vi "readFromXML.vi"(8 "error in (no error)":errorcluster, 11 "file path (use dialog)":path) -> (0 "error out":errorcluster, 3 "Report (Ausgang)":refnum<class "Report.lvclass">)   [LabVIEW 2013, in "XML.lvlib"]
uses:
  lib/XML.lvlib
  classes/Datastructure/Report/Report.lvclass
  classes/Datastructure/Norm/Norm.lvclass
  classes/Datastructure/Test/Test.lvclass
  classes/Datastructure/Image/img.lvclass
  classes/Datastructure/Setup/Setup.lvclass
  classes/Datastructure/Device/Device.lvclass
  <vilib>/xml/Load XML File.vi
  <resource>/objmgr/DOMUserDefRef.rc
  <vilib>/xml/NI_XML.lvlib
panel:
  in  "img id":i32
  out "size(s)":i32
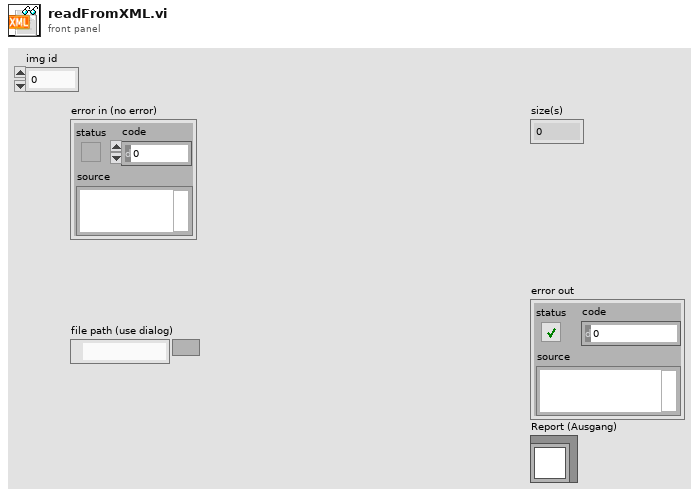
[diagram p1: front panel]
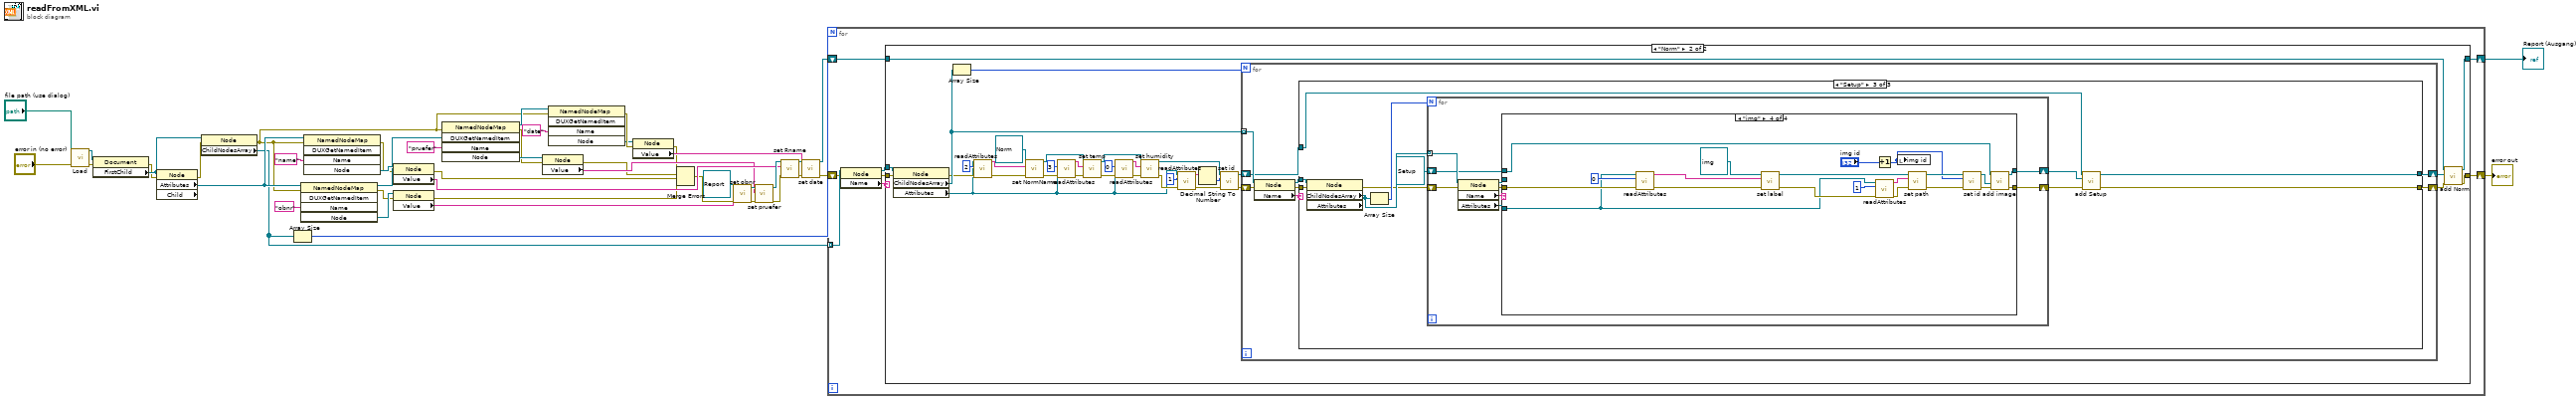
[diagram p0: block diagram]
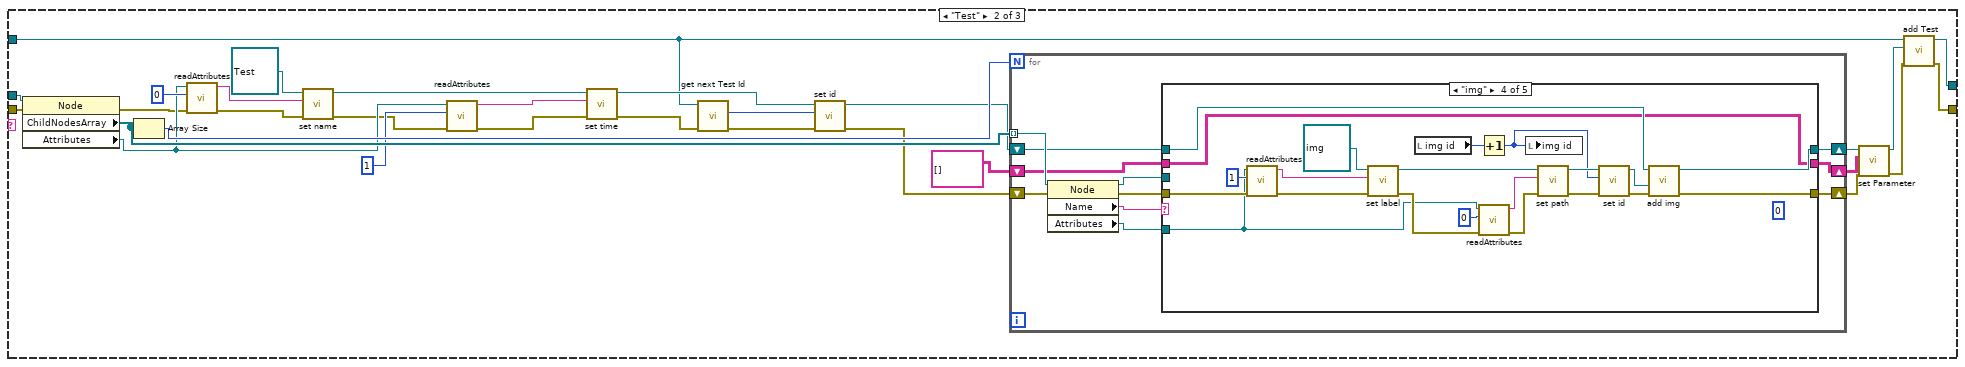
[diagram p4: hidden frame]
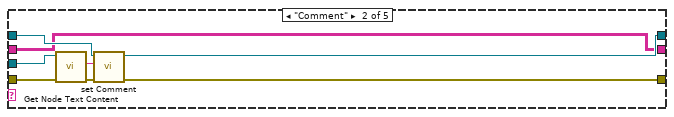
[diagram p6: hidden frame]
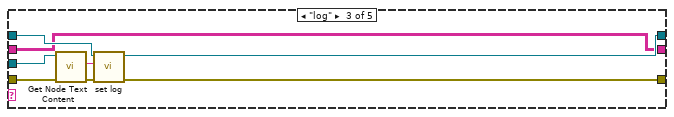
[diagram p7: hidden frame]
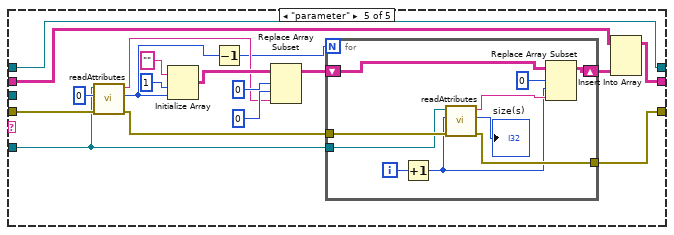
[diagram p8: hidden frame]
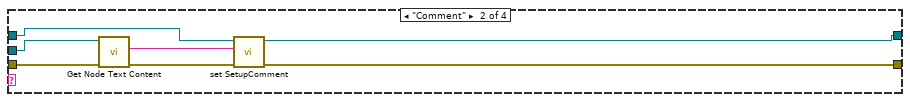
[diagram p10: hidden frame]
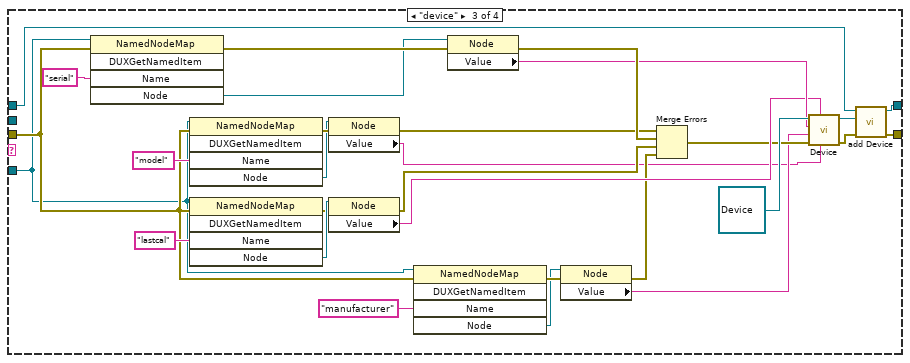
[diagram p11: hidden frame]
diagram:
  n1 = call-poly <vilib>:"Load.vi"("path to XML document"="file path (use dialog)", "error in (no error)"="error in (no error)") -> ("DOM document out"=w42:refnum<k20>, "error out"=w24:errorcluster)  [unwired: 11 in, 1 out]
  n2 = property class="Document"(reference=w42, error in=w24) -> (error out=w23:errorcluster, "FirstChild"=w26:refnum<k20>)  [unwired: 1 out]
  n3 = property class="Node" props=["Attributes", "Child"](reference=w26, error in=w23) -> (error out=w22:errorcluster, "Attributes"=w36:refnum<k20>)  [unwired: 2 out]
  n4 = property on="Eigenschaftsknoten" class="Node"(reference=w26, error in=w22) -> (error out=w2:errorcluster, "ChildNodesArray"=w34:refnum<k20>[])  [unwired: 1 out]
  n5 = Array Size(array=w34) -> (size(s)=w35:i32)
  n6 = invoke class="NamedNodeMap" method="DUXGetNamedItem"(reference=w36, error in=w2, "Name"="obnr") -> (reference out=w38:refnum<k20>, error out=w20:errorcluster, "Node"=w40:refnum<k20>)  [unwired: 2 in, 2 out]
  n7 = invoke class="NamedNodeMap" method="DUXGetNamedItem"(reference=w36, error in=w2, "Name"="name") -> (error out=w21:errorcluster, "Node"=w43:refnum<k20>)  [unwired: 2 in, 3 out]
  n8 = property class="Node"(reference=w43, error in=w21) -> (error out=w3:errorcluster, "Value"=w29:string)  [unwired: 1 out]
  n9 = property class="Node"(reference=w40, error in=w20) -> (error out=w1:errorcluster, "Value"=w30:string)  [unwired: 1 out]
  n10 = invoke class="NamedNodeMap" method="DUXGetNamedItem"(reference=w38, error in=w2, "Name"="pruefer") -> (reference out=w12:refnum<k20>, error out=w19:errorcluster, "Node"=w37:refnum<k20>)  [unwired: 2 in, 2 out]
  n11 = property class="Node"(reference=w37, error in=w19) -> (error out=w4:errorcluster, "Value"=w25:string)  [unwired: 1 out]
  n12 = invoke class="NamedNodeMap" method="DUXGetNamedItem"(reference=w12, error in=w2, "Name"="date") -> (error out=w15:errorcluster, "Node"=w14:refnum<k20>)  [unwired: 2 in, 3 out]
  n13 = property class="Node"(reference=w14, error in=w15) -> (error out=w5:errorcluster, "Value"=w10:string)  [unwired: 1 out]
  n14 = Merge Errors(w5, w4, w3, w1) -> (w6:errorcluster)
  n15 = call-dynamic "set obnr.vi"("error in (no error)"=w6, "obnr"=w30, "Report in"=refnum<class "Report.lvclass"> refnum ("Report.lvclass")) -> ("error out"=w28:errorcluster, "Report out"=w32:refnum<class "Report.lvclass">)  [unwired: 7 in]
  n16 = call-dynamic "set pruefer.vi"("error in (no error)"=w28, "pruefer"=w25, "Report in"=w32) -> ("error out"=w27:errorcluster, "Report out"=w31:refnum<class "Report.lvclass">)  [unwired: 7 in]
  n17 = call-dynamic "set Rname.vi"("error in (no error)"=w27, "Rname"=w29, "Report (Eingang)"=w31) -> ("error out"=w9:errorcluster, "Report (Ausgang)"=w11:refnum<class "Report.lvclass">)  [unwired: 7 in]
  n18 = call-dynamic "set date.vi"("error in (no error)"=w9, "date"=w10, "Report (Eingang)"=w11) -> ("error out"=w8:errorcluster, "Report (Ausgang)"=w7:refnum<class "Report.lvclass">)  [unwired: 7 in]
  n19 = for {
    N: w35 -> [_]
    tunnel: w34 -> [w53] mode=indexing
    shift-right: [w49] -> w17
    shift-left: w7 -> [w51]
    shift-right: [w46] -> w18
    shift-left: w8 -> [w48]
    n20 = property class="Node"(reference=w53, error in=w48) -> (reference out=w50:refnum<k20>, error out=w47:errorcluster, "Name"=w52:string)
    n21 = case shown="\"Norm\"" w52 {
      tunnel: w51 -> [w55 w56]
      tunnel: w50 -> [_ w88]
      tunnel: [w55 w57] -> w49
      tunnel: w47 -> [w54 w81]
      tunnel: [w54 w58] -> w46
      frame "False", Default {
      }
      frame "Norm" {
        n22 = property class="Node"(reference=w88, error in=w81) -> (error out=w74:errorcluster, "ChildNodesArray"=w86:refnum<k20>[], "Attributes"=w62:refnum<k20>)  [unwired: 1 out]
        n23 = Array Size(array=w86) -> (size(s)=w87:i32)
        n24 = call "readAttributes.vi"("Fehler (Eingang, kein Fehler)"=w74, "index"=2, "Refnum in"=w62) -> ("Fehler (Ausgang)"=w73:errorcluster, "Node Value 2"=w83:string)  [unwired: 6 in, 1 out]
        n25 = call-dynamic "set NormName.vi"("error in (no error)"=w73, "name"=w83, "Norm (Eingang)"=refnum<class "Norm.lvclass"> refnum ("Test.lvclass")) -> ("error out"=w72:errorcluster, "Norm (Ausgang)"=w80:refnum<class "Norm.lvclass">)  [unwired: 7 in]
        n26 = call "readAttributes.vi"("Fehler (Eingang, kein Fehler)"=w72, "index"=3, "Refnum in"=w62) -> ("Fehler (Ausgang)"=w71:errorcluster, "Node Value 2"=w76:string)  [unwired: 6 in, 1 out]
        n27 = call-dynamic "set temp.vi"("error in (no error)"=w71, "temp"=w76, "Norm (Eingang)"=w80) -> ("error out"=w70:errorcluster, "Norm (Ausgang)"=w79:refnum<class "Norm.lvclass">)  [unwired: 7 in]
        n28 = call "readAttributes.vi"("Fehler (Eingang, kein Fehler)"=w70, "index"=0, "Refnum in"=w62) -> ("Fehler (Ausgang)"=w69:errorcluster, "Node Value 2"=w75:string)  [unwired: 6 in, 1 out]
        n29 = call-dynamic "set humidity.vi"("error in (no error)"=w69, "humidity"=w75, "Test (Eingang)"=w79) -> ("error out"=w64:errorcluster, "Test (Ausgang)"=w68:refnum<class "Norm.lvclass">)  [unwired: 7 in]
        n30 = call "readAttributes.vi"("Fehler (Eingang, kein Fehler)"=w64, "index"=1, "Refnum in"=w62) -> ("Fehler (Ausgang)"=w63:errorcluster, "Node Value 2"=w66:string)  [unwired: 6 in, 1 out]
        n31 = Decimal String To Number(string=w66) -> (number=w65:i32)  [unwired: 2 in, 1 out]
        n32 = call-dynamic "set id.vi"("error in (no error)"=w63, "id"=w65, "Test (Eingang)"=w68) -> ("error out"=w60:errorcluster, "Test (Ausgang)"=w61:refnum<class "Norm.lvclass">)  [unwired: 7 in]
        n33 = for {
          N: w87 -> [_]
          tunnel: w86 -> [w96] mode=indexing
          shift-right: [w92] -> w82
          shift-left: w61 -> [w93]
          shift-right: [w89] -> w59
          shift-left: w60 -> [w91]
          n34 = property class="Node"(reference=w96, error in=w91) -> (reference out=w94:refnum<k20>, error out=w90:errorcluster, "Name"=w95:string)
          n35 = case shown="\"Setup\"" w95 {
            tunnel: w94 -> [_ w128 w218]
            tunnel: w93 -> [w98 w104 w212]
            tunnel: [w98 w125 w211] -> w92
            tunnel: w90 -> [w97 w118 w215]
            tunnel: [w97 w117 w210] -> w89
            frame "False", Default {
            }
            frame "Test" {
              n36 = property class="Node"(reference=w128, error in=w118) -> (error out=w115:errorcluster, "ChildNodesArray"=w126:refnum<k20>[], "Attributes"=w116:refnum<k20>)  [unwired: 1 out]
              n37 = Array Size(array=w126) -> (size(s)=w127:i32)
              n38 = call "readAttributes.vi"("Fehler (Eingang, kein Fehler)"=w115, "index"=0, "Refnum in"=w116) -> ("Fehler (Ausgang)"=w114:errorcluster, "Node Value 2"=w121:string)  [unwired: 6 in, 1 out]
              n39 = call-dynamic "set name.vi"("error in (no error)"=w114, "name"=w121, "Test (Eingang)"=refnum<class "Test.lvclass"> refnum ("Segment.lvclass")) -> ("error out"=w113:errorcluster, "Test (Ausgang)"=w119:refnum<class "Test.lvclass">)  [unwired: 7 in]
              n40 = call "readAttributes.vi"("Fehler (Eingang, kein Fehler)"=w113, "index"=1, "Refnum in"=w116) -> ("Fehler (Ausgang)"=w112:errorcluster, "Node Value 2"=w122:string)  [unwired: 6 in, 1 out]
              n41 = call-dynamic "set time.vi"("error in (no error)"=w112, "time"=w122, "Test (Eingang)"=w119) -> ("error out"=w103:errorcluster, "Test (Ausgang)"=w105:refnum<class "Test.lvclass">)  [unwired: 7 in]
              n42 = call-dynamic "get next Test Id.vi"("error in (no error)"=w103, "Norm in"=w104) -> ("error out"=w102:errorcluster, "id"=w101:u32)  [unwired: 7 in, 1 out]
              n43 = call-dynamic "set id.vi"("error in (no error)"=w102, "id"=w101, "Test in"=w105) -> ("error out"=w100:errorcluster, "Test out"=w99:refnum<class "Test.lvclass">)  [unwired: 7 in]
              n44 = for {
                N: w127 -> [_]
                tunnel: w126 -> [w139] mode=indexing
                shift-right: [w135] -> w111
                shift-left: w99 -> [w134]
                shift-right: [w131] -> w109
                shift-left: w100 -> [w133]
                shift-right: [w129] -> w110
                shift-left: string[][] [] -> [w130]
                n45 = property class="Node"(reference=w139, error in=w133) -> (reference out=w137:refnum<k20>, error out=w132:errorcluster, "Name"=w138:string, "Attributes"=w136:refnum<k20>)
                n46 = case shown="\"img\"" w138 {
                  tunnel: w137 -> [_ w150 w158 _ _]
                  tunnel: w134 -> [w142 w149 w156 w178 w186]
                  tunnel: w136 -> [_ _ _ w165 w194]
                  tunnel: [w142 w147 w152 w177 w186] -> w135
                  tunnel: w132 -> [w141 w146 w157 w170 w197]
                  tunnel: [w141 w144 w153 w171 w187] -> w131
                  tunnel: [w140 w143 w151 w166 w183] -> w129
                  tunnel: w130 -> [w140 w143 w151 w166 w184]
                  frame "False", Default {
                  }
                  frame "Comment" {
                    n47 = call <vilib>:"Get Node Text Content.vi"("error in (no error)"=w146, "node in"=w150) -> ("error out"=w145:errorcluster, "node text"=w148:string)  [unwired: 7 in, 1 out]
                    n48 = call-dynamic "set Comment.vi"("error in (no error)"=w145, "Comment"=w148, "Test (Eingang)"=w149) -> ("error out"=w144:errorcluster, "Test (Ausgang)"=w147:refnum<class "Test.lvclass">)  [unwired: 7 in]
                  }
                  frame "log" {
                    n49 = call <vilib>:"Get Node Text Content.vi"("error in (no error)"=w157, "node in"=w158) -> ("error out"=w154:errorcluster, "node text"=w155:string)  [unwired: 7 in, 1 out]
                    n50 = call-dynamic "set log.vi"("error in (no error)"=w154, "log"=w155, "Test (Eingang)"=w156) -> ("error out"=w153:errorcluster, "Test (Ausgang)"=w152:refnum<class "Test.lvclass">)  [unwired: 7 in]
                  }
                  frame "img" {
                    (unwired) 0 ("index")
                    n51 = call "readAttributes.vi"("Fehler (Eingang, kein Fehler)"=w170, "index"=1, "Refnum in"=w165) -> ("Fehler (Ausgang)"=w169:errorcluster, "Node Value 2"=w174:string)  [unwired: 6 in, 1 out]
                    n52 = call-dynamic "set label.vi"("error in (no error)"=w169, "label"=w174, "img (Eingang)"=refnum<class "img.lvclass"> refnum ("img.lvclass")) -> ("error out"=w168:errorcluster, "img (Ausgang)"=w172:refnum<class "img.lvclass">)  [unwired: 7 in]
                    n53 = local read "img id"() -> (w160:i32)
                    n54 = Increment(x=w160) -> (x+1=w159:i32)
                    n55 = call "readAttributes.vi"("Fehler (Eingang, kein Fehler)"=w168, "index"=0, "Refnum in"=w165) -> ("Fehler (Ausgang)"=w167:errorcluster, "Node Value 2"=w176:string)  [unwired: 6 in, 1 out]
                    n56 = local write "img id"(w159) -> ()
                    n57 = call-dynamic "set path.vi"("error in (no error)"=w167, "path"=w176, "img (Eingang)"=w172) -> ("error out"=w161:errorcluster, "img (Ausgang)"=w164:refnum<class "img.lvclass">)  [unwired: 7 in]
                    n58 = call-dynamic "set id.vi"("error in (no error)"=w161, "id"=w159, "img in"=w164) -> ("error out"=w163:errorcluster, "img out"=w162:refnum<class "img.lvclass">)  [unwired: 7 in]
                    n59 = call-dynamic "add img.vi"("error in (no error)"=w163, "img.lvclass"=w162, "Test (Eingang)"=w178) -> ("error out"=w171:errorcluster, "Test (Ausgang)"=w177:refnum<class "Test.lvclass">)  [unwired: 6 in]
                  }
                  frame "parameter" {
                    n60 = call "readAttributes.vi"("Fehler (Eingang, kein Fehler)"=w197, "index"=0, "Refnum in"=w194) -> ("Fehler (Ausgang)"=w195:errorcluster, "size(s)"=w180:i32, "Node Value 2"=w188:string)  [unwired: 6 in]
                    n61 = Initialize Array("" ("Element"), 1 ("Dimension"), w180) -> (w191:string[][])
                    n62 = Decrement(x=w180) -> (x-1=w181:i32)
                    n63 = Replace Array Subset(array=w191, new element=w188, index (row)=0 ("Index (Zeile)"), index (col)=0 ("Deaktivierter Index (Spalte)")) -> (w185:string[][])
                    n64 = for {
                      N: w181 -> [_]
                      tunnel: w195 -> [w207]
                      tunnel: w194 -> [w206]
                      tunnel: [w203] -> w187
                      shift-right: [w198] -> w182
                      shift-left: w185 -> [w199]
                      i -> [w202]
                      n65 = Increment(x=w202) -> (x+1=w201:i32)
                      n66 = call "readAttributes.vi"("Fehler (Eingang, kein Fehler)"=w207, "index"=w201, "Refnum in"=w206) -> ("Fehler (Ausgang)"=w203:errorcluster, "size(s)"=→"size(s)":i32, "Node Value 2"=w204:string)  [unwired: 6 in]
                      n67 = Replace Array Subset(array=w199, new element=w204, index (row)=0 ("Index (Zeile)"), index (col)=w201) -> (w198:string[][])
                    }
                    n68 = Insert Into Array(array=w184, new element=w182) -> (w183:string[][])  [unwired: 2 in]
                  }
                }
              }
              n69 = call-dynamic "set Parameter.vi"("error in (no error)"=w109, "Parameter"=w110, "Test (Eingang)"=w111) -> ("error out"=w108:errorcluster, "Test (Ausgang)"=w106:refnum<class "Test.lvclass">)  [unwired: 7 in]
              n70 = call-dynamic "add Test.vi"("error in (no error)"=w108, "Test.lvclass"=w106, "Test Eingang"=w104) -> ("error out"=w117:errorcluster, "Test Ausgang"=w125:refnum<class "Norm.lvclass">)  [unwired: 7 in]
            }
            frame "Setup" {
              n71 = property class="Node" props=["ChildNodesArray", "Attributes"](reference=w218, error in=w215) -> (error out=w213:errorcluster, "ChildNodesArray"=w216:refnum<k20>[])  [unwired: 2 out]
              n72 = Array Size(array=w216) -> (size(s)=w217:i32)
              n73 = for {
                N: w217 -> [_]
                tunnel: w216 -> [w227] mode=indexing
                shift-right: [w223] -> w208
                shift-left: refnum<class "Setup.lvclass"> refnum ("Setup.lvclass") -> [w222]
                shift-right: [w219] -> w209
                shift-left: w213 -> [w221]
                n74 = property class="Node"(reference=w227, error in=w221) -> (reference out=w225:refnum<k20>, error out=w220:errorcluster, "Name"=w226:string, "Attributes"=w224:refnum<k20>)
                n75 = case shown="\"img\"" w226 {
                  tunnel: w225 -> [_ w236 _ _]
                  tunnel: w222 -> [w229 w233 w265 w270]
                  tunnel: w224 -> [_ _ w237 w272]
                  tunnel: [w229 w232 w261 w275] -> w223
                  tunnel: w220 -> [w228 w235 w241 w279]
                  tunnel: [w228 w231 w260 w274] -> w219
                  frame "False", Default {
                  }
                  frame "Comment" {
                    n76 = call <vilib>:"Get Node Text Content.vi"("error in (no error)"=w235, "node in"=w236) -> ("error out"=w230:errorcluster, "node text"=w234:string)  [unwired: 7 in, 1 out]
                    n77 = call-dynamic "set SetupComment.vi"("error in (no error)"=w230, "Comment"=w234, "Setup (Eingang)"=w233) -> ("error out"=w231:errorcluster, "Setup (Ausgang)"=w232:refnum<class "Setup.lvclass">)  [unwired: 7 in]
                  }
                  frame "device" {
                    n78 = invoke class="NamedNodeMap" method="DUXGetNamedItem"(reference=w237, error in=w241, "Name"="serial") -> (error out=w255:errorcluster, "Node"=w252:refnum<k20>)  [unwired: 2 in, 3 out]
                    n79 = invoke class="NamedNodeMap" method="DUXGetNamedItem"(reference=w237, error in=w241, "Name"="model") -> (error out=w259:errorcluster, "Node"=w258:refnum<k20>)  [unwired: 2 in, 3 out]
                    n80 = invoke class="NamedNodeMap" method="DUXGetNamedItem"(reference=w237, error in=w241, "Name"="lastcal") -> (error out=w249:errorcluster, "Node"=w250:refnum<k20>)  [unwired: 2 in, 3 out]
                    n81 = property class="Node"(reference=w258, error in=w259) -> (error out=w253:errorcluster, "Value"=w238:string)  [unwired: 1 out]
                    n82 = property class="Node"(reference=w250, error in=w249) -> (error out=w247:errorcluster, "Value"=w246:string)  [unwired: 1 out]
                    n83 = invoke class="NamedNodeMap" method="DUXGetNamedItem"(reference=w237, error in=w241, "Name"="manufacturer") -> (error out=w243:errorcluster, "Node"=w242:refnum<k20>)  [unwired: 2 in, 3 out]
                    n84 = property class="Node"(reference=w252, error in=w255) -> (error out=w254:errorcluster, "Value"=w251:string)  [unwired: 1 out]
                    n85 = property class="Node"(reference=w242, error in=w243) -> (error out=w240:errorcluster, "Value"=w239:string)  [unwired: 1 out]
                    n86 = Merge Errors(w253, w254, w247, w240) -> (w245:errorcluster)
                    n87 = call-dynamic "Device.vi"("Model"=w238, "last calibration"=w246, "error in (no error)"=w245, "Hersteller"=w239, "serial"=w251, "Device Eingang"=refnum<class "Device.lvclass"> refnum ("Device.lvclass")) -> ("error out"=w262:errorcluster, "Device Ausgang"=w263:refnum<class "Device.lvclass">)  [unwired: 4 in]
                    n88 = call-dynamic "add Device.vi"("error in (no error)"=w262, "Device.lvclass"=w263, "Setup Eingang"=w265) -> ("error out"=w260:errorcluster, "Setup Ausgang"=w261:refnum<class "Setup.lvclass">)  [unwired: 7 in]
                  }
                  frame "img" {
                    n89 = call "readAttributes.vi"("Fehler (Eingang, kein Fehler)"=w279, "index"=0, "Refnum in"=w272) -> ("Fehler (Ausgang)"=w278:errorcluster, "Node Value 2"=w282:string)  [unwired: 6 in, 1 out]
                    n90 = call-dynamic "set label.vi"("error in (no error)"=w278, "label"=w282, "img (Eingang)"=refnum<class "img.lvclass"> refnum ("img.lvclass")) -> ("error out"=w277:errorcluster, "img (Ausgang)"=w280:refnum<class "img.lvclass">)  [unwired: 7 in]
                    n91 = Increment(x="img id") -> (x+1=w266:i32)
                    n92 = call "readAttributes.vi"("Fehler (Eingang, kein Fehler)"=w277, "index"=1, "Refnum in"=w272) -> ("Fehler (Ausgang)"=w276:errorcluster, "Node Value 2"=w284:string)  [unwired: 6 in, 1 out]
                    n93 = local write "img id"(w266) -> ()
                    n94 = call-dynamic "set path.vi"("error in (no error)"=w276, "path"=w284, "img (Eingang)"=w280) -> ("error out"=w268:errorcluster, "img (Ausgang)"=w273:refnum<class "img.lvclass">)  [unwired: 7 in]
                    n95 = call-dynamic "set id.vi"("error in (no error)"=w268, "id"=w266, "img in"=w273) -> ("error out"=w269:errorcluster, "img out"=w271:refnum<class "img.lvclass">)  [unwired: 7 in]
                    n96 = call-dynamic "add image.vi"("error in (no error)"=w269, "img.lvclass"=w271, "Setup (Eingang)"=w270) -> ("error out"=w274:errorcluster, "Setup (Ausgang)"=w275:refnum<class "Setup.lvclass">)  [unwired: 7 in]
                  }
                }
              }
              n97 = call-dynamic "add Setup.vi"("error in (no error)"=w209, "Setup"=w208, "Test Eingang"=w212) -> ("error out"=w210:errorcluster, "Test Ausgang"=w211:refnum<class "Norm.lvclass">)  [unwired: 7 in]
            }
          }
        }
        n98 = call-dynamic "add Norm.vi"("error in (no error)"=w59, "Norm.lvclass"=w82, "Report (Eingang)"=w56) -> ("error out"=w58:errorcluster, "Report (Ausgang)"=w57:refnum<class "Report.lvclass">)  [unwired: 7 in]
      }
    }
  }
  "error out" <- w18
  "Report (Ausgang)" <- w17
